vi "kvCanGetVersionEx.vi"(2 "error in (no error)":errorcluster, 3 "Version Type":u32(ring) items=["DLL Version", "DLL Product Version"]) -> (0 "error out":errorcluster, 1 "Version (hex)":u16 format="%.0x")   [LabVIEW 2022 SP3]
doc: "This function returns various version numbers from the driver routines."
uses:
  canlib32.dll
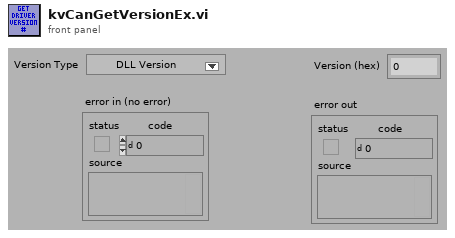
[diagram p1: front panel]
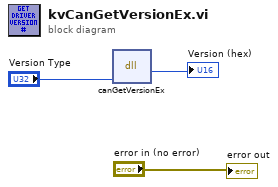
[diagram p0: block diagram]
diagram:
  n1 = dll-call lib="canlib32.dll" fn="canGetVersionEx"("itemCode"="Version Type") -> (→"Version (hex)":u16)  [unwired: 4 in, 2 out]
  "error out" <- "error in (no error)"
